vi "OpenArm.vi"(7 "Wrist PID":T1={"No Bin"={"P"=30.0, "I"=0.0, "D"=100.0}, "Bin"={"P"=0.0, "I"=0.0, "D"=0.0}}, 8 "error in (no error)":errorcluster, 10 "Pivot PID":T1={"No Bin"={"P"=15.0, "I"=0.0, "D"=0.0}, "Bin"={"P"=15.0, "I"=0.0, "D"=0.0}}, 11 "Extension PID":T1={"No Bin"={"P"=40.0, "I"=0.0, "D"=0.0}, "Bin"={"P"=0.0, "I"=0.0, "D"=0.0}}) -> (0 "error out":errorcluster)   [LabVIEW 2015]
uses:
  <vilib>/Rock Robotics/WPI/CAN/TalonSRX/WPI_CANTalonSRX_APIControlMode.ctl
  <vilib>/Rock Robotics/WPI/CAN/TalonSRX/WPI_CANTalonSRX_APIFeedbackSelect.ctl
  Robot Global Data.vi
  <vilib>/Rock Robotics/WPI/MotorControl/WPI_MotorControlOpenCANTalonSRX.vi
panel:
  in  "Reverse Pivot Limit":dbl
  in  "Forward Pivot Limit":dbl=512.0
  in  "Reverse Claw Limit":dbl=64.0 format="%#_13g"
  in  "Forward Claw Limit":dbl=215.0 format="%#_13g"
  in  "Forward Wrist Limit":dbl=256.0
  in  "Reverse Wrist Limit":dbl=-256.0
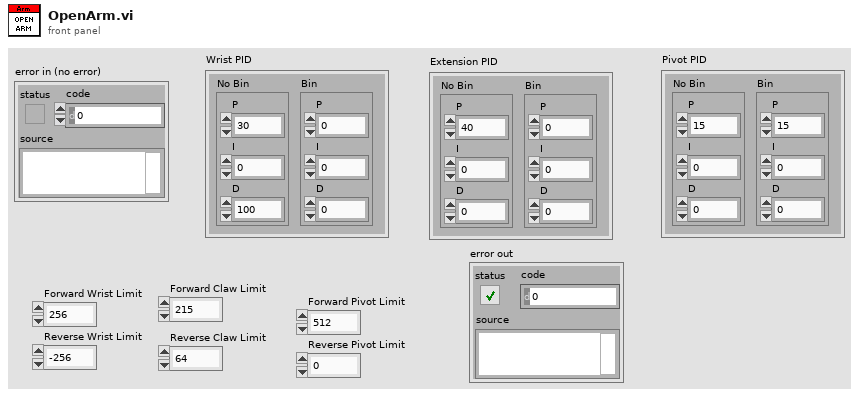
[diagram p1: front panel]
types:
  T1 = cluster{"No Bin":cluster{"P":dbl, "I":dbl, "D":dbl}, "Bin":cluster{"P":dbl, "I":dbl, "D":dbl}}
  T2 = typedef "WPI_CANTalonSRX_APIControlMode.ctl" = enum8{"Percent VBus", "Speed", "Position", "Slave", "Unchanged / Invalid"}
  T3 = typedef "WPI_CANTalonSRX_APIFeedbackSelect.ctl" = enum16{"Digital Quadrature Encoder", "Analog Potentiometer", "Analog Encoder"}
  T4 = typedef "WPI_MotorControlDeviceRef.ctl" = cluster{"DeviceStatus":errorcluster, "Type":T5, "PWM":cluster{"PWM Channel":T6, "DeadBand":T7}, "CAN":cluster{"Device Number":u8, "Control Mode":T8, "Semaphore":T9, "Max Vout":dbl, "TalonSRX Control Mode":T2}, "Invert":bool, "TransformRef":T10, "InvTransformRef":T10}
  T5 = typedef "WPI_MotorControlType.ctl" = enum16{"PWM", "CAN", "CANTalonSRX"}
  T6 = typedef "FPGA_DIOPWMChannel.ctl" = enum8{"PWM 0", "PWM 1", "PWM 2", "PWM 3", "PWM 4", "PWM 5", "PWM 6", "PWM 7", "PWM 8", "PWM 9", "PWM MXP 0", "PWM MXP 1", "PWM MXP 2", "PWM MXP 3", "PWM MXP 4", "PWM MXP 5", "PWM MXP 6", "PWM MXP 7", "PWM MXP 8", "PWM MXP 9", "Invalid"}
  T7 = typedef "WPI_PWMDeadband.ctl" = cluster{"Name":string, "maxPositivePwm":i32, "minPositivePwm":i32, "centerPwm":i32, "maxNegativePwm":i32, "minNegativePwm":i32, "angularRange":u16}
  T8 = typedef "WPI_CANJaguar_ControlMode.ctl" = enum8{"Percent VBus", "Current", "Speed", "Position", "Voltage"}
  T9 = typedef "Semaphore RefNum" = refnum<k1>
  T10 = typedef "WPI_PWMTransform_ConPane.ctl" = refnum<vi>
  T11 = typedef "WPI_CANTalonSRX_GlobalStatus.ctl" = cluster{"Applied Throttle":dbl, "Module Enabled":bool, "CAN Error":errorcluster, "Closed Loop Error":dbl, "Forward Limit Switch Closed":bool, "Reverse Limit Switch Closed":bool, "Sensor Position":dbl, "Sensor Velocity":dbl, "Current":dbl, "Sticky Fault - Over Temp":bool, "Sticky Fault - Under Voltage":bool, "Sticky Fault - Forward Limit":bool, "Sticky Fault - Reverse Limit":bool, "Sticky Fault - Forward Soft Limit":bool, "Sticky Fault - Reverse Soft Limit":bool, "Brake is Enabled":bool, "Encoder Position":dbl, "Encoder Velocity":dbl, "Encoder Index Count":dbl, "Encoder A Pin State":bool, "Encoder B Pin State":bool, "Encoder Index Pin State":bool, "Analog In":dbl, "Analog In Velocity":dbl, "Temperature (C)":dbl, "Battery Voltage":dbl}
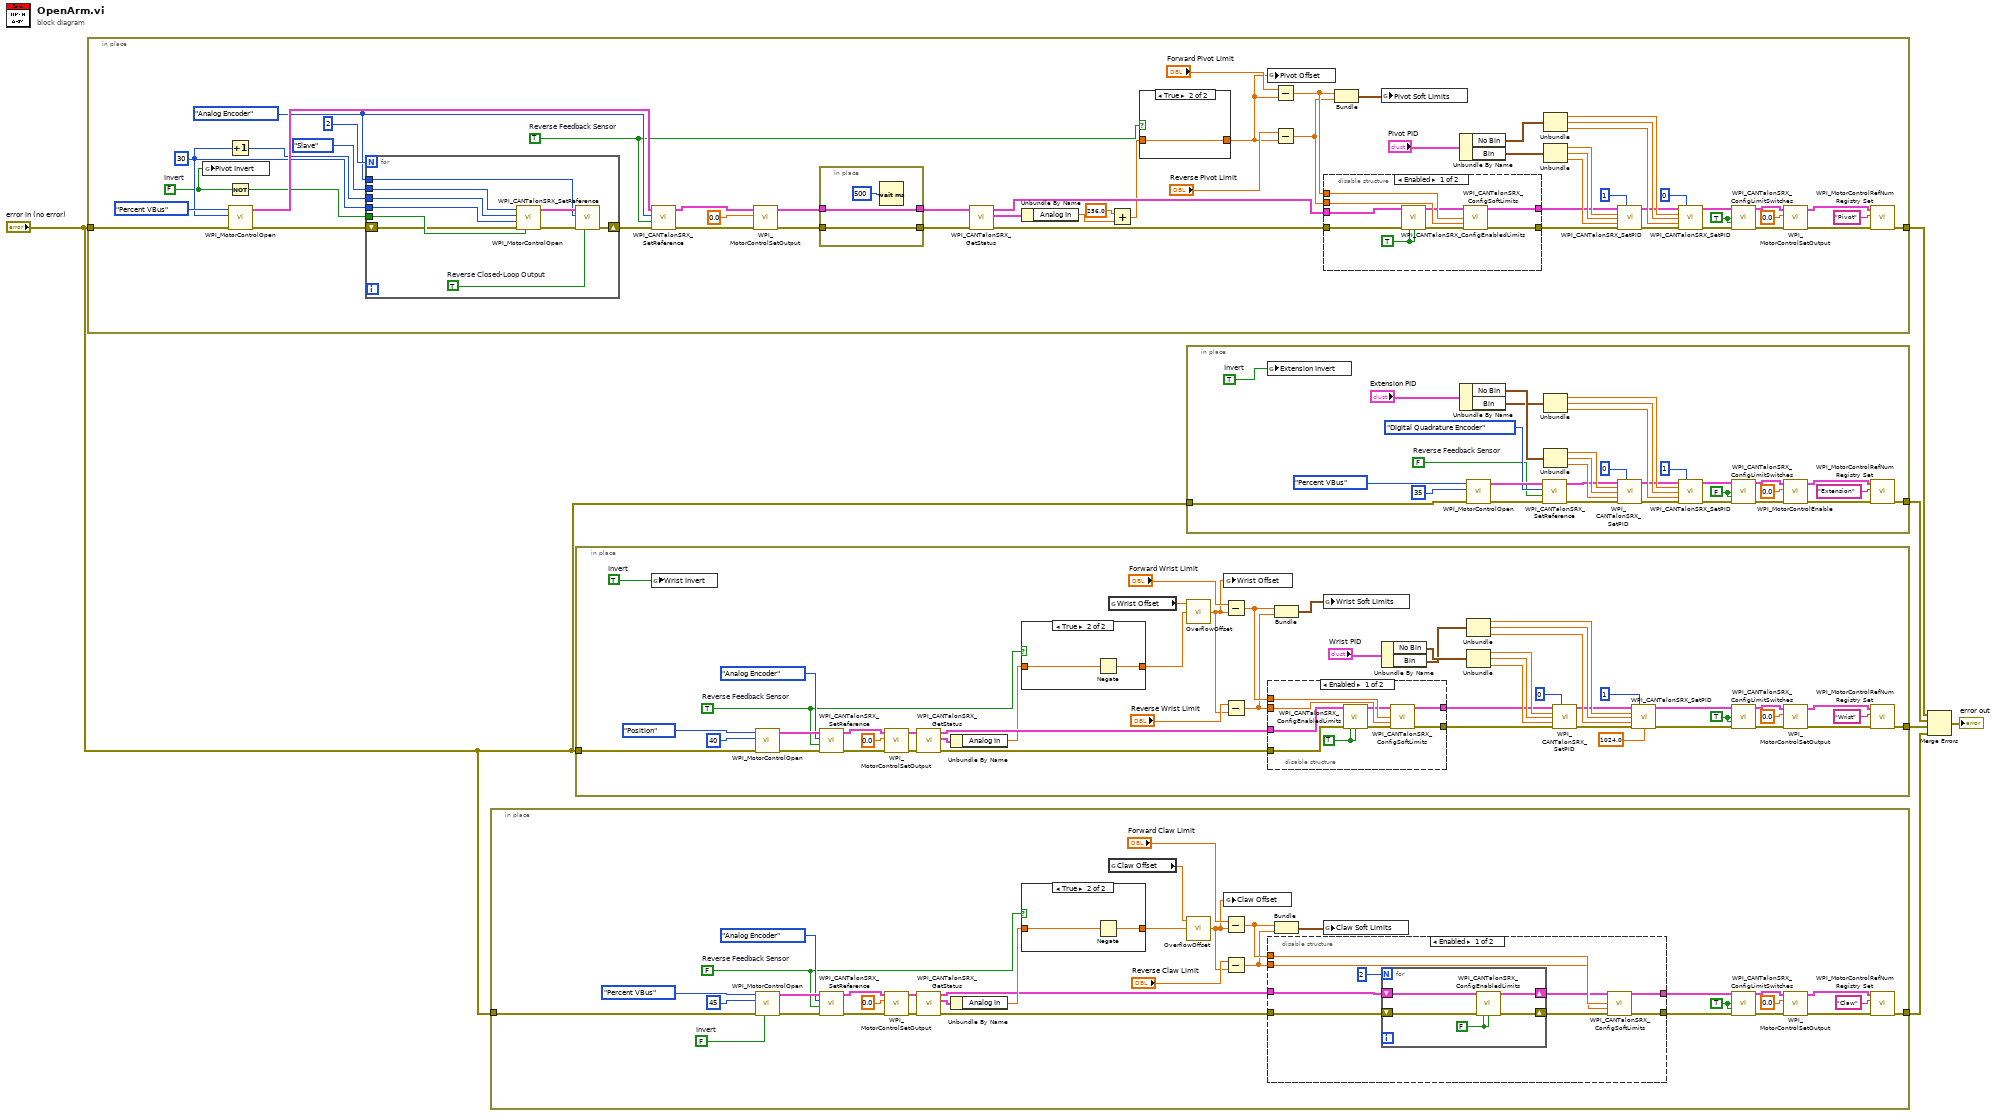
[diagram p0: block diagram]
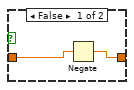
[diagram p4: hidden frame]
diagram:
  n1 = in-place {
    in-place-border: [w60] -> w6
    in-place-border: "error in (no error)" -> [w59]
    w21 = TRUE  # Reverse Feedback Sensor
    w20 = FALSE  # Invert
    w57 = TRUE ("Forward Limit Switch Normally Open")
    w40 = WPI_CANTalonSRX_APIFeedbackSelect."Analog Encoder" ("Feedback Reference")
    w44 = u8 30 ("Pivot ID")
    n2 = global write "Robot Global Data.vi" "Pivot Invert"(w20) -> ()
    n3 = Increment(x=w44) -> (x+1=w46:u8)
    n4 = Not(x=w20) -> (.not. x?=w45:bool)
    n5 = call-poly <vilib>:"WPI_MotorControlOpen.vi"("error in (no error)"=w59, "Device Number"=w44, "Control Mode"=WPI_CANTalonSRX_APIControlMode."Percent VBus") -> ("error out"=w43:errorcluster, "MotorControlDeviceRef"=w58:T4)  [unwired: 7 in]
    n6 = for {
      N: 2 -> [_]
      tunnel: WPI_CANTalonSRX_APIControlMode."Slave" ("Control Mode") -> [w79]
      tunnel: w46 -> [w78]
      tunnel: w45 -> [w77]
      tunnel: w44 -> [w76]
      shift-right: [w72] -> w42
      shift-left: w43 -> [w75]
      tunnel: w40 -> [w71]
      w70 = TRUE  # Reverse Closed-Loop Output
      n7 = call-poly <vilib>:"WPI_MotorControlOpen.vi"("Invert"=w77, "error in (no error)"=w75, "Master Device Number"=w76, "Device Number"=w78, "Control Mode"=w79) -> ("error out"=w73:errorcluster, "MotorControlDeviceRef"=w74:T4)  [unwired: 5 in]
      n8 = call <vilib>:"WPI_CANTalonSRX_SetReference.vi"("Reverse Closed-Loop Output"=w70, "error in (no error)"=w73, "Feedback Reference"=w71, "CAN Talon SRX Ref"=w74) -> ("error out"=w72:errorcluster)  [unwired: 6 in, 1 out]
    }
    n9 = call <vilib>:"WPI_CANTalonSRX_SetReference.vi"("error in (no error)"=w42, "Reverse Feedback Sensor"=w21, "Feedback Reference"=w40, "CAN Talon SRX Ref"=w58) -> ("error out"=w10:errorcluster, "CAN Talon SRX Ref"=w11:T4)  [unwired: 6 in]
    n10 = call <vilib>:"WPI_MotorControlSetOutput.vi"("error in (no error)"=w10, "Output"=0.0 ("Analog In"), "MotorControlDevRef"=w11) -> ("error out"=w8:errorcluster, "MotorControlDevRef"=w9:T4)  [unwired: 6 in, 1 out]
    n11 = in-place {
      in-place-border: [w65] -> w14
      in-place-border: w9 -> [w65]
      in-place-border: [w64] -> w13
      in-place-border: w8 -> [w64]
      n12 = Wait (ms)(milliseconds to wait=u32 500) -> ()  [unwired: 1 out]
    }
    n13 = call <vilib>:"WPI_CANTalonSRX_GetStatus.vi"("error in (no error)"=w13, "CAN Talon SRX Ref"=w14) -> ("error out"=w27:errorcluster, "Talon SRX Status"=w25:T11, "CAN Talon SRX Ref"=w26:T4)  [unwired: 7 in]
    n14 = Unbundle By Name(w25) -> ("Analog In"=w7:dbl)
    n15 = Add(x=256.0, y=w7) -> (x+y=w22:dbl)
    n16 = case shown="True" w21 {
      tunnel: [w67 w69] -> w23
      tunnel: w22 -> [w68 w69]
      frame False {
        n17 = Negate(x=w68) -> (-x=w67:dbl)
      }
      frame True {
      }
    }
    n18 = global write "Robot Global Data.vi" "Pivot Offset"(w23) -> ()
    n19 = Subtract(x="Forward Pivot Limit", y=w23) -> (x-y=w52:dbl)
    n20 = Subtract(x="Reverse Pivot Limit", y=w23) -> (x-y=w51:dbl)
    n21 = disable-structure shown="Enabled" {
      disable-tunnel: w26 -> [w84 w90]
      disable-tunnel: w27 -> [w85 w89]
      disable-tunnel: w52 -> [w88 _]
      disable-tunnel: w51 -> [w87 _]
      disable-tunnel: [w82 w89] -> w50
      disable-tunnel: [w80 w90] -> w49
      frame Enabled {
        w86 = TRUE ("Forward Soft Limit Enable")
        n22 = call <vilib>:"WPI_CANTalonSRX_ConfigEnabledLimits.vi"("CAN Talon SRX Ref"=w84, "error in (no error)"=w85, "Forward Soft Limit Enable"=w86, "Reverse Soft Limit Enable"=w86) -> ("CAN Talon SRX Ref"=w81:T4, "error out"=w83:errorcluster)  [unwired: 10 in]
        n23 = call <vilib>:"WPI_CANTalonSRX_ConfigSoftLimits.vi"("CAN Talon SRX Ref"=w81, "Forward Limit Position"=w88, "Reverse Limit Position"=w87, "error in (no error)"=w83) -> ("CAN Talon SRX Ref"=w80:T4, "error out"=w82:errorcluster)  [unwired: 10 in]
      }
      frame Disabled {
      }
    }
    n24 = Bundle(w52, w51) -> (w53:cluster{dbl, dbl})  [unwired: 1 in]
    n25 = global write "Robot Global Data.vi" "Pivot Soft Limits"(w53) -> ()
    n26 = Unbundle By Name("Pivot PID") -> ("No Bin"=w32:cluster{"P":dbl, "I":dbl, "D":dbl}, "Bin"=w31:cluster{"P":dbl, "I":dbl, "D":dbl})
    n27 = Unbundle(w32) -> ("P"=w37:dbl, "I"=w38:dbl, "D"=w39:dbl)
    n28 = Unbundle(w31) -> ("P"=w61:dbl, "I"=w62:dbl, "D"=w63:dbl)
    n29 = call <vilib>:"WPI_CANTalonSRX_SetPID.vi"("CAN Talon SRX Ref"=w49, "Parameter Slot"=u8 1, "P"=w61, "I"=w62, "D"=w63, "error in (no error)"=w50) -> ("CAN Talon SRX Ref Out"=w35:T4, "error out"=w34:errorcluster)  [unwired: 8 in]
    n30 = call <vilib>:"WPI_CANTalonSRX_SetPID.vi"("CAN Talon SRX Ref"=w35, "Parameter Slot"=u8 0, "P"=w37, "I"=w38, "D"=w39, "error in (no error)"=w34) -> ("CAN Talon SRX Ref Out"=w30:T4, "error out"=w29:errorcluster)  [unwired: 8 in]
    n31 = call <vilib>:"WPI_CANTalonSRX_ConfigLimitSwitches.vi"("CAN Talon SRX Ref"=w30, "Forward Limit Switch Normally Open"=w57, "Reverse Limit Switch Normally Open"=w57, "error in (no error)"=w29) -> ("CAN Talon SRX Ref"=w18:T4, "error out"=w17:errorcluster)  [unwired: 10 in]
    n32 = call <vilib>:"WPI_MotorControlSetOutput.vi"("error in (no error)"=w17, "Output"=0.0 ("Analog In"), "MotorControlDevRef"=w18) -> ("error out"=w16:errorcluster, "MotorControlDevRef"=w15:T4)  [unwired: 6 in, 1 out]
    n33 = call <vilib>:"WPI_MotorControlRefNum Registry Set.vi"("error in (no error)"=w16, "refnum name"="Pivot", "MotorControlDevRef"=w15) -> ("error out"=w60:errorcluster)  [unwired: 7 in, 1 out]
  }
  n34 = in-place {
    in-place-border: [w122] -> w2
    in-place-border: "error in (no error)" -> [w121]
    w91 = FALSE  # Reverse Feedback Sensor
    w118 = TRUE ("Forward Limit Switch Normally Open")
    w109 = FALSE  # Invert
    n35 = call-poly <vilib>:"WPI_MotorControlOpen.vi"("Invert"=w109, "error in (no error)"=w121, "Device Number"=u8 45 ("Claw ID"), "Control Mode"=WPI_CANTalonSRX_APIControlMode."Percent VBus") -> ("error out"=w112:errorcluster, "MotorControlDeviceRef"=w120:T4)  [unwired: 6 in]
    n36 = call <vilib>:"WPI_CANTalonSRX_SetReference.vi"("error in (no error)"=w112, "Reverse Feedback Sensor"=w91, "Feedback Reference"=WPI_CANTalonSRX_APIFeedbackSelect."Analog Encoder", "CAN Talon SRX Ref"=w120) -> ("error out"=w98:errorcluster, "CAN Talon SRX Ref"=w97:T4)  [unwired: 6 in]
    n37 = call <vilib>:"WPI_MotorControlSetOutput.vi"("error in (no error)"=w98, "Output"=0.0 ("Analog In"), "MotorControlDevRef"=w97) -> ("error out"=w101:errorcluster, "MotorControlDevRef"=w102:T4)  [unwired: 6 in, 1 out]
    n38 = call <vilib>:"WPI_CANTalonSRX_GetStatus.vi"("error in (no error)"=w101, "CAN Talon SRX Ref"=w102) -> ("error out"=w95:errorcluster, "Talon SRX Status"=w100:T11, "CAN Talon SRX Ref"=w96:T4)  [unwired: 7 in]
    n39 = Unbundle By Name(w100) -> ("Analog In"=w99:dbl)
    n40 = case shown="True" w91 {
      tunnel: w99 -> [w126 w128]
      tunnel: [w126 w127] -> w92
      frame False {
      }
      frame True {
        n41 = Negate(x=w128) -> (-x=w127:dbl)
      }
    }
    n42 = global read "Robot Global Data.vi" "Claw Offset"() -> (w94:dbl)
    n43 = call "OverflowOffset.vi"("Sensor Position"=w92, "Current Offset"=w94) -> ("New Offset"=w93:dbl)  [unwired: 3 in]
    n44 = global write "Robot Global Data.vi" "Claw Offset"(w93) -> ()
    n45 = Subtract(x="Forward Claw Limit", y=w93) -> (x-y=w114:dbl)
    n46 = Subtract(x="Reverse Claw Limit", y=w93) -> (x-y=w113:dbl)
    n47 = disable-structure shown="Enabled" {
      disable-tunnel: w114 -> [w137 _]
      disable-tunnel: w113 -> [w136 _]
      disable-tunnel: [w135 w143] -> w111
      disable-tunnel: [w134 w144] -> w110
      disable-tunnel: w96 -> [w133 w144]
      disable-tunnel: w95 -> [w132 w143]
      frame Enabled {
        n48 = for {
          N: 2 -> [_]
          shift-right: [w139] -> w131
          shift-left: w133 -> [w141]
          shift-right: [w138] -> w130
          shift-left: w132 -> [w140]
          w142 = FALSE ("Forward Soft Limit Enable")
          n49 = call <vilib>:"WPI_CANTalonSRX_ConfigEnabledLimits.vi"("CAN Talon SRX Ref"=w141, "error in (no error)"=w140, "Forward Soft Limit Enable"=w142, "Reverse Soft Limit Enable"=w142) -> ("CAN Talon SRX Ref"=w139:T4, "error out"=w138:errorcluster)  [unwired: 10 in]
        }
        n50 = call <vilib>:"WPI_CANTalonSRX_ConfigSoftLimits.vi"("CAN Talon SRX Ref"=w131, "Forward Limit Position"=w137, "Reverse Limit Position"=w136, "error in (no error)"=w130) -> ("CAN Talon SRX Ref"=w134:T4, "error out"=w135:errorcluster)  [unwired: 10 in]
      }
      frame Disabled {
      }
    }
    n51 = Bundle(w114, w113) -> (w115:cluster{dbl, dbl})  [unwired: 1 in]
    n52 = global write "Robot Global Data.vi" "Claw Soft Limits"(w115) -> ()
    n53 = call <vilib>:"WPI_CANTalonSRX_ConfigLimitSwitches.vi"("CAN Talon SRX Ref"=w110, "Forward Limit Switch Normally Open"=w118, "Reverse Limit Switch Normally Open"=w118, "error in (no error)"=w111) -> ("CAN Talon SRX Ref"=w108:T4, "error out"=w107:errorcluster)  [unwired: 10 in]
    n54 = call <vilib>:"WPI_MotorControlSetOutput.vi"("error in (no error)"=w107, "Output"=0.0, "MotorControlDevRef"=w108) -> ("error out"=w106:errorcluster, "MotorControlDevRef"=w105:T4)  [unwired: 6 in, 1 out]
    n55 = call <vilib>:"WPI_MotorControlRefNum Registry Set.vi"("error in (no error)"=w106, "refnum name"="Claw", "MotorControlDevRef"=w105) -> ("error out"=w122:errorcluster)  [unwired: 7 in, 1 out]
  }
  n56 = in-place {
    in-place-border: [w190] -> w4
    in-place-border: "error in (no error)" -> [w189]
    w145 = TRUE  # Reverse Feedback Sensor
    w184 = TRUE ("Forward Limit Switch Normally Open")
    w163 = TRUE  # Invert
    n57 = global write "Robot Global Data.vi" "Wrist Invert"(w163) -> ()
    n58 = call-poly <vilib>:"WPI_MotorControlOpen.vi"("error in (no error)"=w189, "Device Number"=u8 40 ("Wrist ID"), "Control Mode"=WPI_CANTalonSRX_APIControlMode."Position") -> ("error out"=w187:errorcluster, "MotorControlDeviceRef"=w188:T4)  [unwired: 7 in]
    n59 = call <vilib>:"WPI_CANTalonSRX_SetReference.vi"("error in (no error)"=w187, "Reverse Feedback Sensor"=w145, "Feedback Reference"=WPI_CANTalonSRX_APIFeedbackSelect."Analog Encoder", "CAN Talon SRX Ref"=w188) -> ("error out"=w153:errorcluster, "CAN Talon SRX Ref"=w154:T4)  [unwired: 6 in]
    n60 = call <vilib>:"WPI_MotorControlSetOutput.vi"("error in (no error)"=w153, "Output"=0.0 ("Analog In"), "MotorControlDevRef"=w154) -> ("error out"=w155:errorcluster, "MotorControlDevRef"=w156:T4)  [unwired: 6 in, 1 out]
    n61 = call <vilib>:"WPI_CANTalonSRX_GetStatus.vi"("error in (no error)"=w155, "CAN Talon SRX Ref"=w156) -> ("error out"=w151:errorcluster, "Talon SRX Status"=w150:T11, "CAN Talon SRX Ref"=w152:T4)  [unwired: 7 in]
    n62 = Unbundle By Name(w150) -> ("Analog In"=w149:dbl)
    n63 = case shown="True" w145 {
      tunnel: w149 -> [w196 w198]
      tunnel: [w196 w197] -> w146
      frame False {
      }
      frame True {
        n64 = Negate(x=w198) -> (-x=w197:dbl)
      }
    }
    n65 = global read "Robot Global Data.vi" "Wrist Offset"() -> (w148:dbl)
    n66 = call "OverflowOffset.vi"("Sensor Position"=w146, "Current Offset"=w148) -> ("New Offset"=w147:dbl)  [unwired: 3 in]
    n67 = global write "Robot Global Data.vi" "Wrist Offset"(w147) -> ()
    n68 = Subtract(x="Forward Wrist Limit", y=w147) -> (x-y=w182:dbl)
    n69 = Subtract(x="Reverse Wrist Limit", y=w147) -> (x-y=w181:dbl)
    n70 = disable-structure shown="Enabled" {
      disable-tunnel: w151 -> [w200 w208]
      disable-tunnel: w152 -> [w199 w209]
      disable-tunnel: w182 -> [w207 _]
      disable-tunnel: w181 -> [w206 _]
      disable-tunnel: [w203 w209] -> w180
      disable-tunnel: [w204 w208] -> w179
      frame Enabled {
        w205 = TRUE ("Forward Soft Limit Enable")
        n71 = call <vilib>:"WPI_CANTalonSRX_ConfigEnabledLimits.vi"("CAN Talon SRX Ref"=w199, "error in (no error)"=w200, "Forward Soft Limit Enable"=w205, "Reverse Soft Limit Enable"=w205) -> ("CAN Talon SRX Ref"=w202:T4, "error out"=w201:errorcluster)  [unwired: 10 in]
        n72 = call <vilib>:"WPI_CANTalonSRX_ConfigSoftLimits.vi"("CAN Talon SRX Ref"=w202, "Forward Limit Position"=w207, "Reverse Limit Position"=w206, "error in (no error)"=w201) -> ("CAN Talon SRX Ref"=w203:T4, "error out"=w204:errorcluster)  [unwired: 10 in]
      }
      frame Disabled {
      }
    }
    n73 = Bundle(w182, w181) -> (w183:cluster{dbl, dbl})  [unwired: 1 in]
    n74 = global write "Robot Global Data.vi" "Wrist Soft Limits"(w183) -> ()
    n75 = Unbundle By Name("Wrist PID") -> ("No Bin"=w166:cluster{"P":dbl, "I":dbl, "D":dbl}, "Bin"=w165:cluster{"P":dbl, "I":dbl, "D":dbl})
    n76 = Unbundle(w165) -> ("P"=w173:dbl, "I"=w174:dbl, "D"=w175:dbl)
    n77 = Unbundle(w166) -> ("P"=w191:dbl, "I"=w192:dbl, "D"=w193:dbl)
    n78 = call <vilib>:"WPI_CANTalonSRX_SetPID.vi"("CAN Talon SRX Ref"=w180, "Parameter Slot"=u8 0, "P"=w191, "I"=w192, "D"=w193, "error in (no error)"=w179) -> ("CAN Talon SRX Ref Out"=w171:T4, "error out"=w170:errorcluster)  [unwired: 8 in]
    n79 = call <vilib>:"WPI_CANTalonSRX_SetPID.vi"("CAN Talon SRX Ref"=w171, "Parameter Slot"=u8 1, "P"=w173, "I"=w174, "D"=w175, "error in (no error)"=w170, "I Zone"=1024.0) -> ("CAN Talon SRX Ref Out"=w169:T4, "error out"=w168:errorcluster)  [unwired: 7 in]
    n80 = call <vilib>:"WPI_CANTalonSRX_ConfigLimitSwitches.vi"("CAN Talon SRX Ref"=w169, "Forward Limit Switch Normally Open"=w184, "Reverse Limit Switch Normally Open"=w184, "error in (no error)"=w168) -> ("CAN Talon SRX Ref"=w160:T4, "error out"=w161:errorcluster)  [unwired: 10 in]
    n81 = call <vilib>:"WPI_MotorControlSetOutput.vi"("error in (no error)"=w161, "Output"=0.0, "MotorControlDevRef"=w160) -> ("error out"=w158:errorcluster, "MotorControlDevRef"=w159:T4)  [unwired: 6 in, 1 out]
    n82 = call <vilib>:"WPI_MotorControlRefNum Registry Set.vi"("error in (no error)"=w158, "refnum name"="Wrist", "MotorControlDevRef"=w159) -> ("error out"=w190:errorcluster)  [unwired: 7 in, 1 out]
  }
  n83 = in-place {
    in-place-border: [w238] -> w5
    in-place-border: "error in (no error)" -> [w237]
    w228 = FALSE  # Reverse Feedback Sensor
    w229 = FALSE ("Forward Limit Switch Normally Open")
    w210 = TRUE  # Invert
    n84 = global write "Robot Global Data.vi" "Extension Invert"(w210) -> ()
    n85 = Unbundle By Name("Extension PID") -> ("No Bin"=w221:cluster{"P":dbl, "I":dbl, "D":dbl}, "Bin"=w211:cluster{"P":dbl, "I":dbl, "D":dbl})
    n86 = call-poly <vilib>:"WPI_MotorControlOpen.vi"("error in (no error)"=w237, "Device Number"=u8 35 ("Extension ID"), "Control Mode"=WPI_CANTalonSRX_APIControlMode."Percent VBus") -> ("error out"=w232:errorcluster, "MotorControlDeviceRef"=w235:T4)  [unwired: 7 in]
    n87 = call <vilib>:"WPI_CANTalonSRX_SetReference.vi"("error in (no error)"=w232, "Reverse Feedback Sensor"=w228, "Feedback Reference"=WPI_CANTalonSRX_APIFeedbackSelect."Digital Quadrature Encoder", "CAN Talon SRX Ref"=w235) -> ("error out"=w233:errorcluster, "CAN Talon SRX Ref"=w234:T4)  [unwired: 6 in]
    n88 = Unbundle(w211) -> ("P"=w217:dbl, "I"=w218:dbl, "D"=w219:dbl)
    n89 = Unbundle(w221) -> ("P"=w239:dbl, "I"=w240:dbl, "D"=w241:dbl)
    n90 = call <vilib>:"WPI_CANTalonSRX_SetPID.vi"("CAN Talon SRX Ref"=w234, "Parameter Slot"=u8 0, "P"=w239, "I"=w240, "D"=w241, "error in (no error)"=w233) -> ("CAN Talon SRX Ref Out"=w215:T4, "error out"=w214:errorcluster)  [unwired: 8 in]
    n91 = call <vilib>:"WPI_CANTalonSRX_SetPID.vi"("CAN Talon SRX Ref"=w215, "Parameter Slot"=u8 1, "P"=w217, "I"=w218, "D"=w219, "error in (no error)"=w214) -> ("CAN Talon SRX Ref Out"=w213:T4, "error out"=w212:errorcluster)  [unwired: 8 in]
    n92 = call <vilib>:"WPI_CANTalonSRX_ConfigLimitSwitches.vi"("CAN Talon SRX Ref"=w213, "Forward Limit Switch Normally Open"=w229, "Reverse Limit Switch Normally Open"=w229, "error in (no error)"=w212) -> ("CAN Talon SRX Ref"=w223:T4, "error out"=w224:errorcluster)  [unwired: 10 in]
    n93 = call <vilib>:"WPI_MotorControlEnable.vi"("error in (no error)"=w224, "Encoder Initial Position"=0.0 ("Analog In"), "CAN Jaguar Ref"=w223) -> ("error out"=w226:errorcluster, "CAN Jaguar Ref"=w227:T4)  [unwired: 7 in]
    n94 = call <vilib>:"WPI_MotorControlRefNum Registry Set.vi"("error in (no error)"=w226, "refnum name"="Extension", "MotorControlDevRef"=w227) -> ("error out"=w238:errorcluster)  [unwired: 7 in, 1 out]
  }
  n95 = Merge Errors(w6, w5, w4, w2) -> (→"error out":errorcluster)
